vi "Get Short Class Name.vi"(4 "KObject in":refnum<class "KObject.lvclass">) -> (1 "Class":string)   [LabVIEW 2020, in "KObject.lvclass"]
uses:
  KObject.lvclass
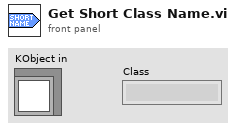
[diagram p1: front panel]
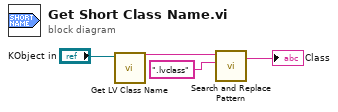
[diagram p0: block diagram]
diagram:
  n1 = call <vilib>:"Get LV Class Name.vi"("object"="KObject in") -> ("class name"=w3:string)  [unwired: 9 in, 1 out]
  n2 = call <vilib>:"Search and Replace Pattern.vi"("string"=w3, "regular expression (\"\")"=".lvclass" ("regular expression (\"\")")) -> ("result string"=→"Class":string)  [unwired: 3 in, 1 out]
